vi "BusOut_write.vi"(8 "error in (no error)":errorcluster, 10 "value":dbl, 11 "BusOut in":refnum<class "BusOut.lvclass">) -> (0 "error out":errorcluster, 3 "BusOut out":refnum<class "BusOut.lvclass">)   [LabVIEW 2011, in "mbed_LVLibrary.lvlib" / "BusOut.lvclass"]
uses:
  BusOut.lvclass
  BusOut.lvclass/BusOut.ctl
  Transport Mechanisms/mbed/mbed.lvclass
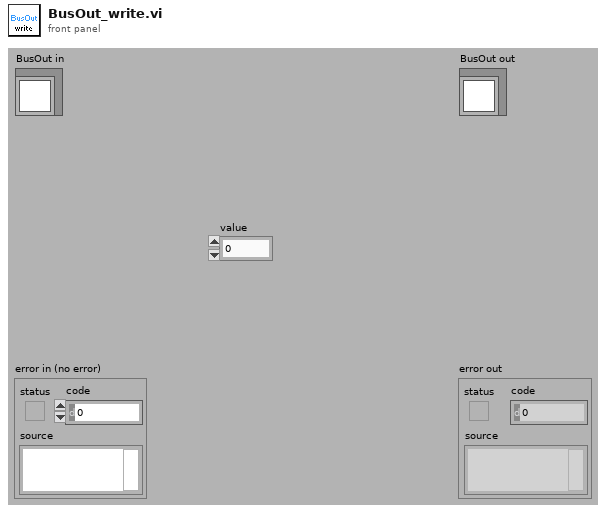
[diagram p1: front panel]
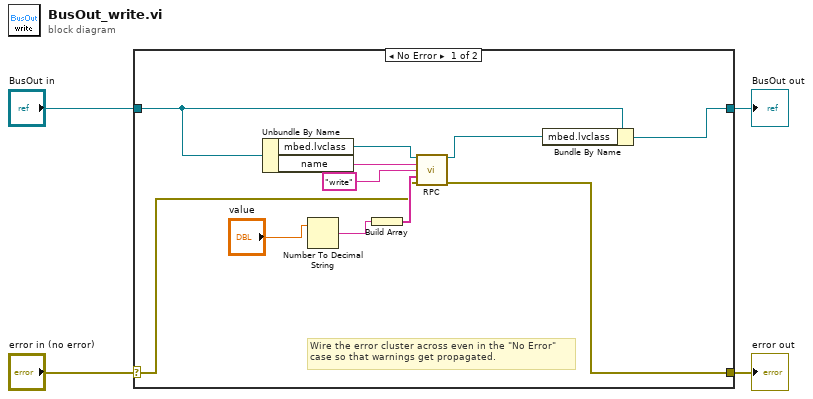
[diagram p0: block diagram]
diagram:
  n1 = case shown="No Error" "error in (no error)" {
    selector: "error in (no error)" -> [w6 w17]
    tunnel: [w5 w17] -> w3
    tunnel: [w14 w16] -> w1
    tunnel: "BusOut in" -> [w15 w16]
    frame No Error {
      # "Wire the error cluster across even in the \"No Error\"\ncase so that warnings get propagated."
      n2 = Unbundle By Name(w15) -> ("mbed.lvclass"=w13:refnum<class "mbed.lvclass">, "name"=w11:string)
      n3 = Number To Decimal String(number="value") -> (decimal integer string=w7:string)  [unwired: 1 in]
      n4 = Build Array(w7) -> (w8:string[])
      n5 = call-dynamic "RPC.vi"("mbed in"=w13, "Name"=w11, "method"="write", "Args"=w8, "error in (no error)"=w6) -> ("mbed out"=w12:refnum<class "mbed.lvclass">, "error out"=w5:errorcluster)  [unwired: 8 in, 1 out]
      n6 = Bundle By Name(cluster=w15, "mbed.lvclass"=w12) -> (w14:refnum<class "BusOut.lvclass">)
    }
    frame Error {
    }
  }
  "error out" <- w3
  "BusOut out" <- w1
